vi "GetVIDesactivationEvent.vi"(8 "error in (no error)":errorcluster, 11 "VI Activation in":refnum<class "VIActivation.lvclass">) -> (0 "error out":errorcluster, 2 "VIDesactivation":refnum<user-event>, 3 "VI Activation out":refnum<class "VIActivation.lvclass">)   [LabVIEW 2021, in "VIActivation.lvlib" / "VIActivation.lvclass"]
uses:
  VIActivation.lvclass
  VIActivation.lvclass/VIActivation.ctl
  VIActivationEvents.ctl
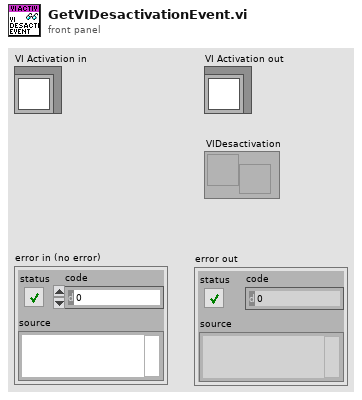
[diagram p1: front panel]
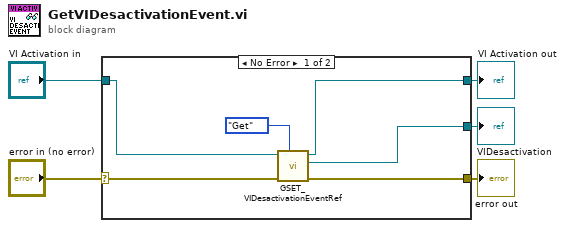
[diagram p0: block diagram]
diagram:
  n1 = case shown="No Error" "error in (no error)" {
    selector: "error in (no error)" -> [w11 w12]
    tunnel: [w8 _] -> w1
    tunnel: "VI Activation in" -> [w7 w13]
    tunnel: [w10 w12] -> w4
    tunnel: [w6 w13] -> w2
    frame No Error {
      n2 = call "GSET_VIDesactivationEventRef.vi"("Action"=enum16{"Get", "Set"}."Get", "error in (no error)"=w11, "VI Activation in"=w7) -> ("error out"=w10:errorcluster, "VIDesactivationEvent out"=w8:refnum<user-event>, "VI Activation out"=w6:refnum<class "VIActivation.lvclass">)  [unwired: 6 in]
    }
    frame Error {
    }
  }
  "VI Activation out" <- w2
  "error out" <- w4
  "VIDesactivation" <- w1
